vi "get v list.vi"(8 "temp":dbl=300.0, 9 "increase":dbl=50.0 format="%#_13g", 10 "end":dbl=144.0 format="%#_13g", 11 "begin":dbl=-72.0 format="%#_13g") -> (0 "输出数组":dbl[](array[numeric]))   [LabVIEW 2019]
uses:
  63af7802-b27c-445f-a4b1-73af5a0d4bd6.vi
panel:
  out "数组":dbl[](array[numeric])
  out "数组 2":dbl[](array[numeric])
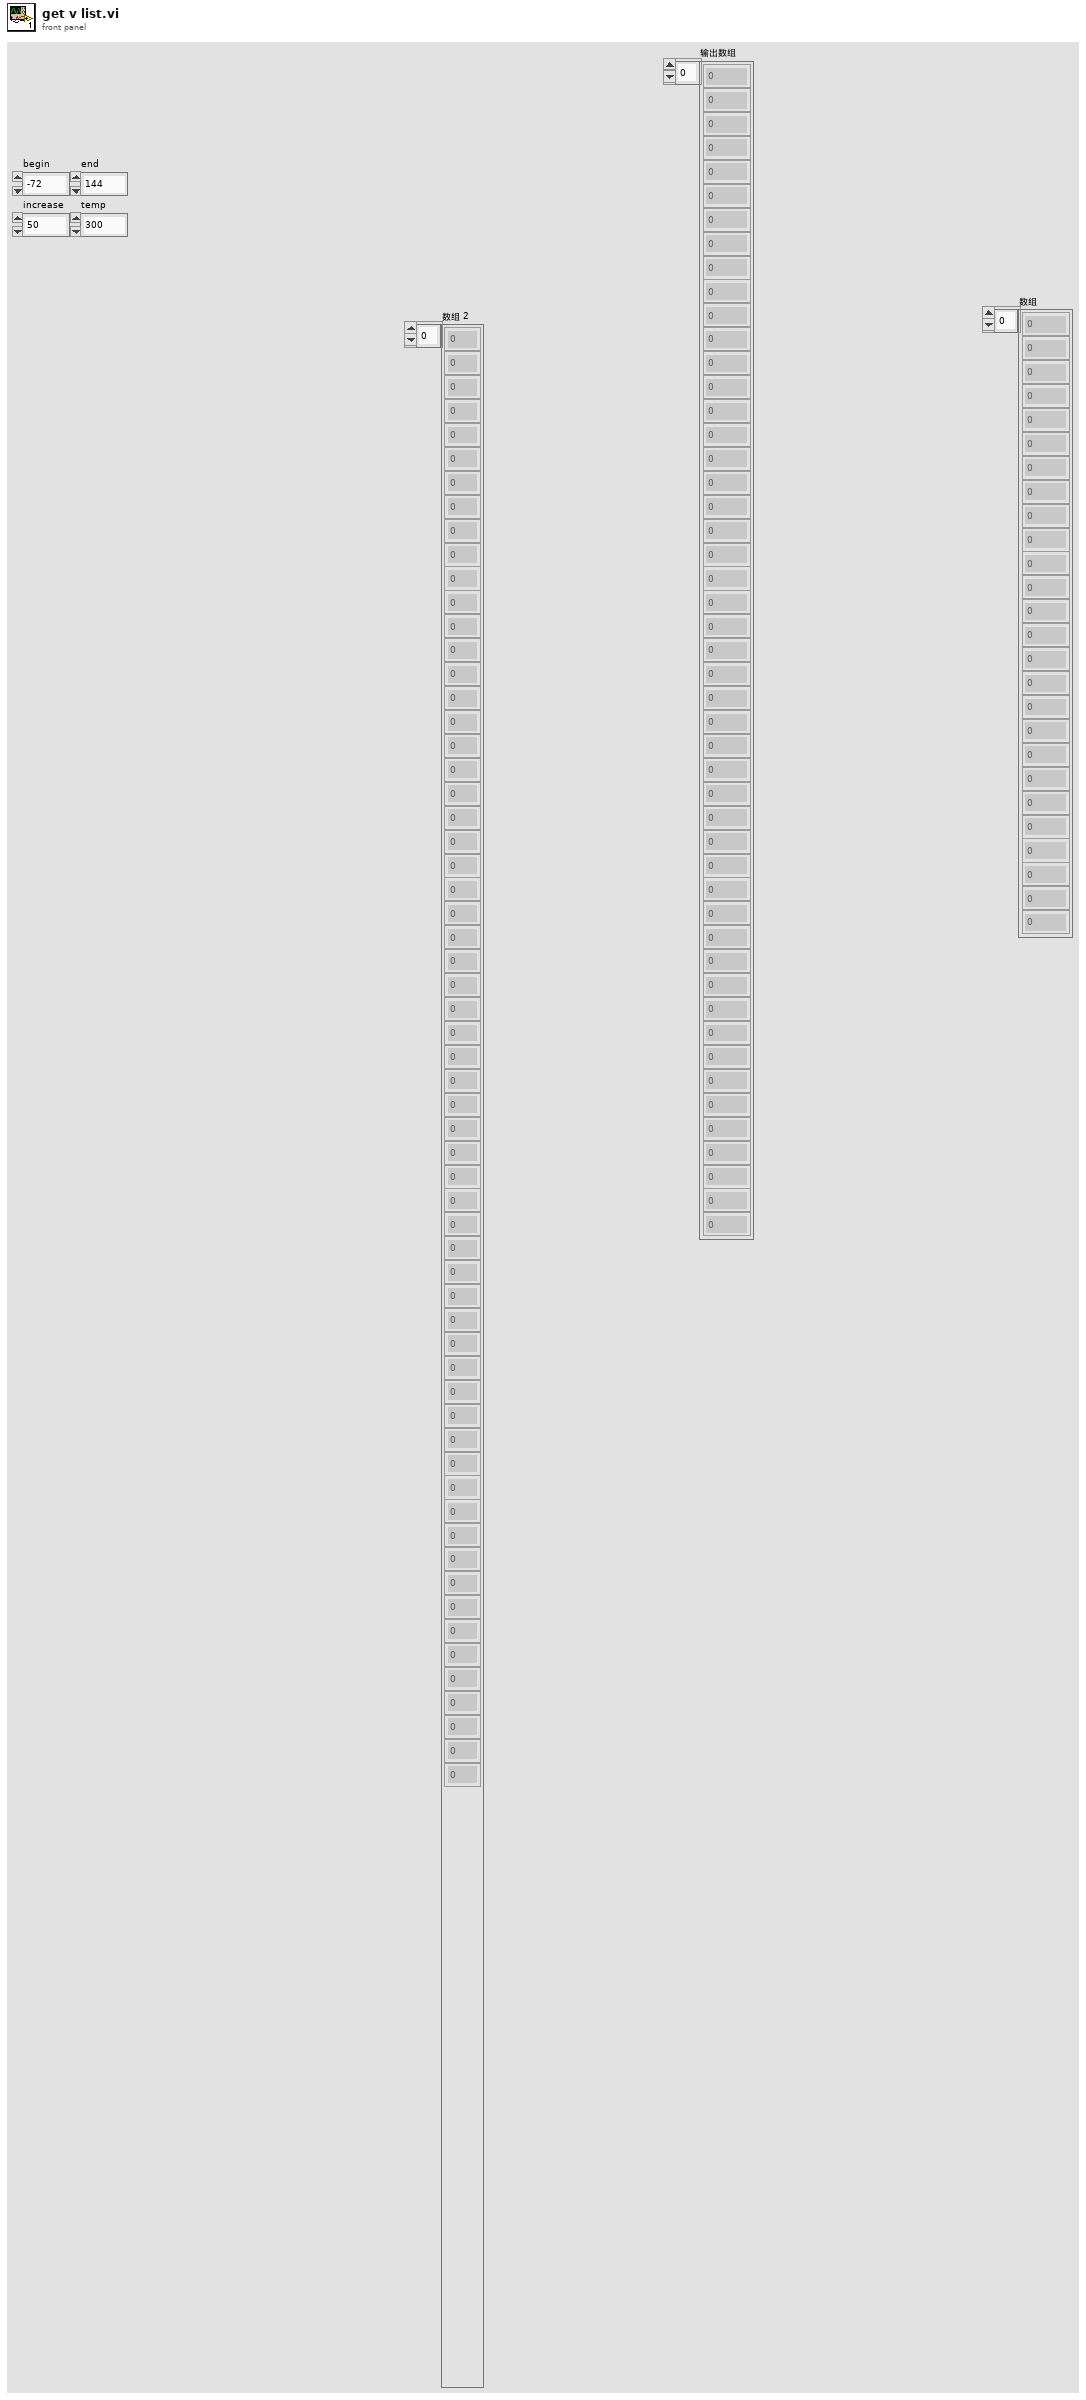
[diagram p1: front panel]
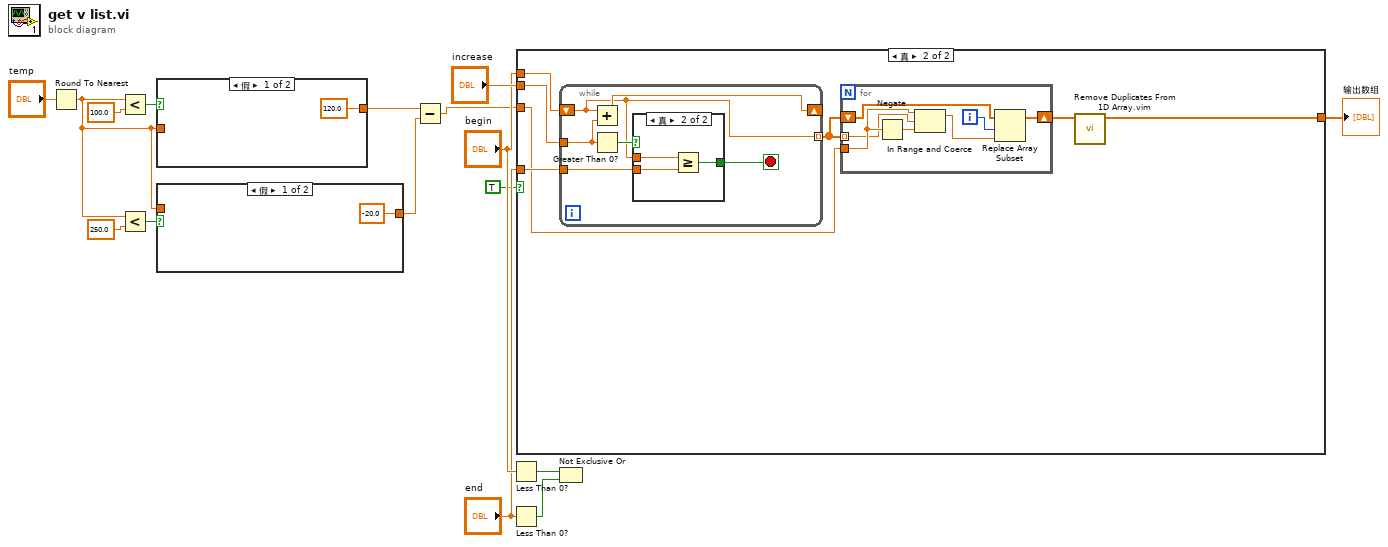
[diagram p0: block diagram]
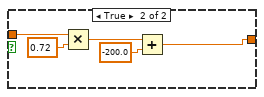
[diagram p2: hidden frame]
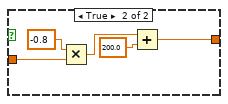
[diagram p3: hidden frame]
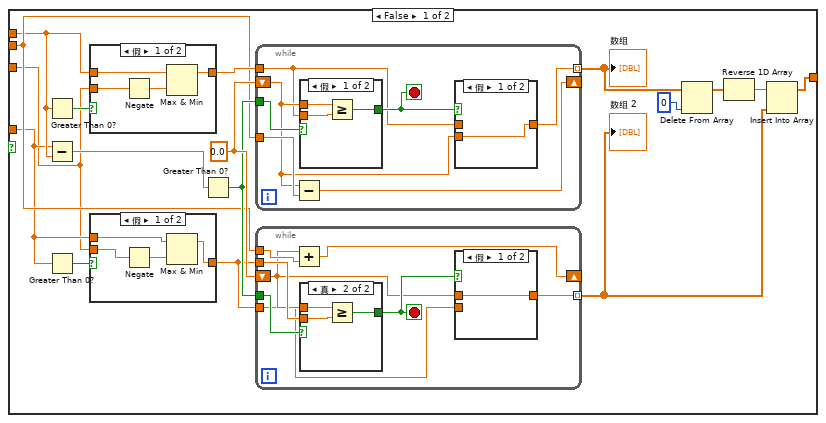
[diagram p4: hidden frame]
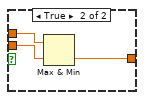
[diagram p5: hidden frame]
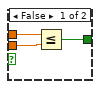
[diagram p7: hidden frame]
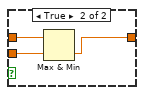
[diagram p8: hidden frame]
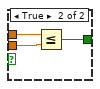
[diagram p10: hidden frame]
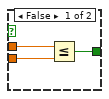
[diagram p11: hidden frame]
diagram:
  n1 = Round To Nearest(number="temp") -> (nearest integer value=w8:dbl)
  n2 = Less?(x=w8, y=100.0) -> (x < y?=w6:bool)
  n3 = Less?(x=w8, y=250.0) -> (x < y?=w7:bool)
  n4 = case shown="假" w6 {
    tunnel: w8 -> [_ w19]
    tunnel: [120.0 w18] -> w9
    frame False {
    }
    frame True {
      n5 = Multiply(x=-0.8, y=w19) -> (x*y=w21:dbl)
      n6 = Add(x=w21, y=200.0) -> (x+y=w18:dbl)
    }
  }
  n7 = case shown="假" w7 {
    tunnel: w8 -> [_ w28]
    tunnel: [-20.0 w24] -> w10
    frame False {
    }
    frame True {
      n8 = Multiply(x=w28, y=0.72) -> (x*y=w26:dbl)
      n9 = Add(x=w26, y=-200.0) -> (x+y=w24:dbl)
    }
  }
  n10 = Subtract(x=w9, y=w10) -> (x-y=w2:dbl)
  n11 = Less Than 0?(x="begin") -> (x < 0?=w11:bool)
  n12 = Less Than 0?(x="end") -> (x < 0?=w12:bool)
  n13 = case shown="真" TRUE {
    tunnel: "increase" -> [w33 w97]
    tunnel: "begin" -> [w32 w96]
    tunnel: "end" -> [w31 w95]
    tunnel: [w30 w91] -> w13
    tunnel: w2 -> [w29 w94]
    frame False {
      w42 = 0.0
      n14 = Greater Than 0?(x=w32) -> (x > 0?=w44:bool)
      n15 = Subtract(x=w31, y=w32) -> (x-y=w45:dbl)
      n16 = Greater Than 0?(x=w31) -> (x > 0?=w40:bool)
      n17 = case shown="假" w44 {
        tunnel: w32 -> [w72 w75]
        tunnel: w29 -> [w70 w74]
        tunnel: [w71 w73] -> w43
        frame False {
          n18 = Negate(x=w70) -> (-x=w69:dbl)
          n19 = Max & Min(x=w72, y=w69) -> (max(x,y)=w71:dbl)  [unwired: 1 out]
        }
        frame True {
          n20 = Max & Min(x=w75, y=w74) -> (min(x,y)=w73:dbl)  [unwired: 1 out]
        }
      }
      n21 = case shown="假" w40 {
        tunnel: w31 -> [w49 w52]
        tunnel: w29 -> [w47 w51]
        tunnel: [w48 w50] -> w34
        frame False {
          n22 = Negate(x=w47) -> (-x=w46:dbl)
          n23 = Max & Min(x=w49, y=w46) -> (max(x,y)=w48:dbl)  [unwired: 1 out]
        }
        frame True {
          n24 = Max & Min(x=w52, y=w51) -> (min(x,y)=w50:dbl)  [unwired: 1 out]
        }
      }
      n25 = Greater Than 0?(x=w45) -> (x > 0?=w41:bool)
      n26 = while {
        tunnel: w33 -> [w80]
        shift-right: [w81] -> _
        shift-left: w42 -> [w78]
        tunnel: w43 -> [w77]
        tunnel: w41 -> [w82]
        tunnel: [w76] -> w39 mode=indexing
        stop <- w79 stop-if-true
        n27 = Subtract(x=w78, y=w80) -> (x-y=w81:dbl)
        n28 = case shown="假" w82 {
          tunnel: w78 -> [w87 w90]
          tunnel: w77 -> [w86 w89]
          tunnel: [w85 w88] -> w79
          frame False {
            n29 = Greater Or Equal?(x=w87, y=w86) -> (x >= y?=w85:bool)
          }
          frame True {
            n30 = Less Or Equal?(x=w90, y=w89) -> (x <= y?=w88:bool)
          }
        }
        n31 = case shown="假" w79 {
          tunnel: [w83 w84] -> w76
          tunnel: w78 -> [w83 _]
          tunnel: w77 -> [_ w84]
          frame False {
          }
          frame True {
          }
        }
      }
      "数组" <- w39
      n32 = while {
        tunnel: w33 -> [w60]
        shift-right: [w57] -> _
        shift-left: w42 -> [w55]
        tunnel: w34 -> [w58]
        tunnel: w41 -> [w59]
        tunnel: [w53] -> w35 mode=indexing
        tunnel: w34 -> [w54]
        stop <- w56 stop-if-true
        n33 = Add(x=w55, y=w60) -> (x+y=w57:dbl)
        n34 = case shown="真" w59 {
          tunnel: w55 -> [w65 w68]
          tunnel: w58 -> [w64 w67]
          tunnel: [w63 w66] -> w56
          frame False {
            n35 = Less Or Equal?(x=w65, y=w64) -> (x <= y?=w63:bool)
          }
          frame True {
            n36 = Greater Or Equal?(x=w68, y=w67) -> (x >= y?=w66:bool)
          }
        }
        n37 = case shown="假" w56 {
          tunnel: w55 -> [w61 _]
          tunnel: [w61 w62] -> w53
          tunnel: w54 -> [_ w62]
          frame False {
          }
          frame True {
          }
        }
      }
      "数组 2" <- w35
      n38 = Delete From Array(array=w39, index=0 ("索引")) -> (array with subset deleted=w37:dbl[])  [unwired: 1 in, 1 out]
      n39 = Reverse 1D Array(array=w37) -> (reversed array=w36:dbl[])
      n40 = Insert Into Array(array=w36, new element=w35) -> (w30:dbl[])  [unwired: 1 in]
    }
    frame True {
      n41 = while {
        tunnel: w97 -> [w110]
        shift-right: [w108] -> _
        shift-left: w96 -> [w105]
        tunnel: w95 -> [w107]
        tunnel: [w105] -> w93 mode=indexing
        stop <- w106 stop-if-true
        n42 = Add(x=w105, y=w110) -> (x+y=w108:dbl)
        n43 = Greater Than 0?(x=w110) -> (x > 0?=w109:bool)
        n44 = case shown="真" w109 {
          tunnel: w105 -> [w113 w116]
          tunnel: w107 -> [w112 w115]
          tunnel: [w111 w114] -> w106
          frame False {
            n45 = Less Or Equal?(x=w113, y=w112) -> (x <= y?=w111:bool)
          }
          frame True {
            n46 = Greater Or Equal?(x=w116, y=w115) -> (x >= y?=w114:bool)
          }
        }
      }
      n47 = for {
        tunnel: w94 -> [w104]
        tunnel: w93 -> [w102] mode=indexing
        shift-right: [w99] -> w92
        shift-left: w93 -> [w101]
        i -> [w98]
        n48 = Negate(x=w104) -> (-x=w103:dbl)
        n49 = In Range and Coerce(upper limit=w104, x=w102, lower limit=w103) -> (coerced(x)=w100:dbl)  [unwired: 1 out]
        n50 = Replace Array Subset(array=w101, new element=w100, index=w98) -> (w99:dbl[])
      }
      n51 = call "Remove Duplicates From 1D Array.vim"("array"=w92) -> ("array with duplicates removed"=w91:dbl[])  [unwired: 10 in]
    }
  }
  "输出数组" <- w13
  n52 = Not Exclusive Or(1:w12, 2:w11) -> ()  [unwired: 1 out]
